vi "Graphics-Defer Panel Updates.vi"(0 "VI":refnum<vi>, 7 "Defer (F)":bool, 11 "error in (no error)":errorcluster) -> (4 "VI out":refnum<vi>, 15 "error out":errorcluster)   [LabVIEW 2020]
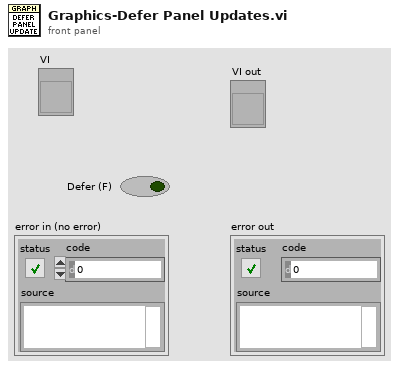
[diagram p1: front panel]
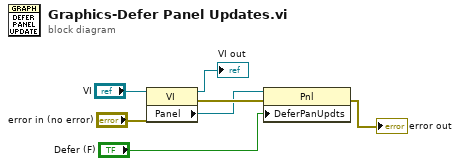
[diagram p0: block diagram]
diagram:
  n1 = property class="VI"(reference="VI", error in="error in (no error)") -> (reference out=→"VI out":refnum<vi>, error out=w6:errorcluster, "Panel"=w1:refnum<vi>)
  n2 = property class="Pnl"(reference=w1, error in=w6, "DeferPanUpdts"="Defer (F)") -> (error out=→"error out":errorcluster)  [unwired: 1 out]
